vi "Edit_Raw_data_file_setups.vi"(4 "LDA set up":T1={"dimensions"=enum."2D", "Arrival spacing"=FALSE, "Sigma cut"=6, "Transit time"=FALSE, "Min time interval ms"=0.1} {"Min time interval ms" format="%.1f"}, 5 "LDA stats weighting":string, 6 "Raw data filename":path, 7 "Meas setup file":string="Colourimeter setup") -> ()   [LabVIEW 2010]
uses:
  Globals/Constants_global.vi
panel:
  out "Appended string":string
  out "Output string":string
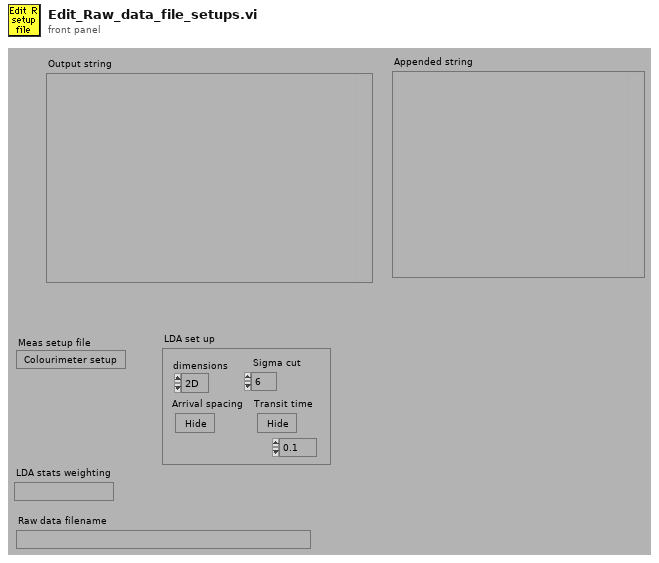
[diagram p1: front panel]
types:
  T1 = cluster{"dimensions":enum16{"1D", "2D"}, "Arrival spacing":bool, "Sigma cut":i32, "Transit time":bool, "Min time interval ms":dbl}
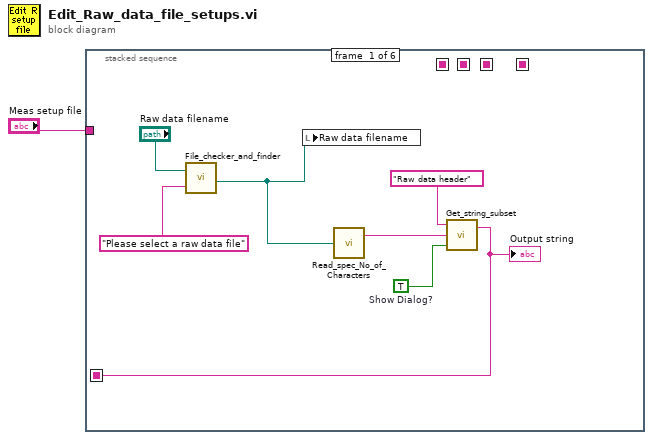
[diagram p0: block diagram]
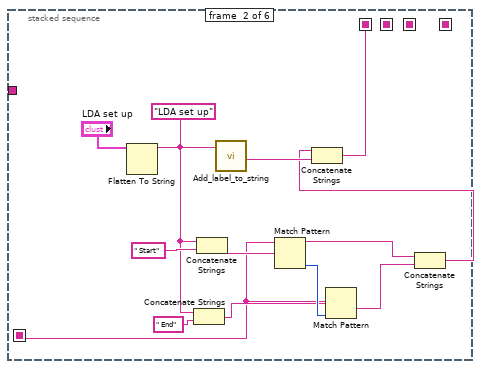
[diagram p2: hidden frame]
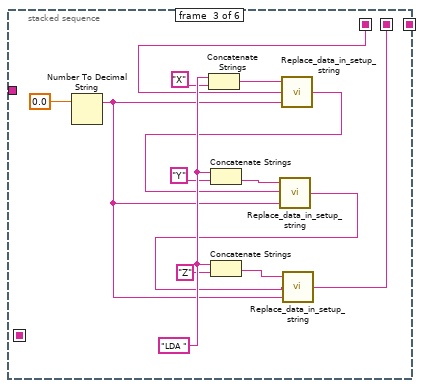
[diagram p3: hidden frame]
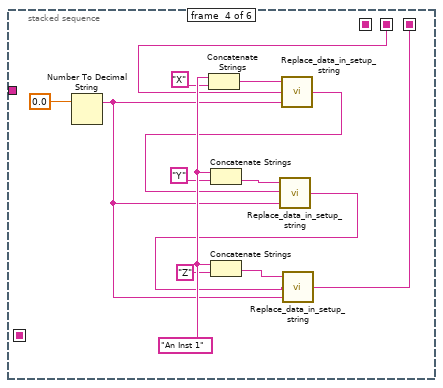
[diagram p4: hidden frame]
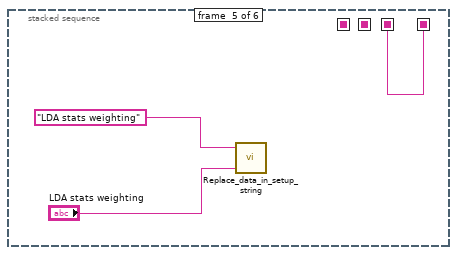
[diagram p5: hidden frame]
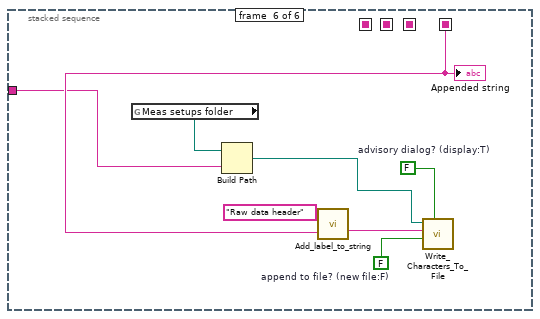
[diagram p6: hidden frame]
diagram:
  n1 = stacked-sequence {
    seq-local: [w7 _ _ _ _ _] -> [_ w12 _ _ _ _]
    seq-local: [_ _ _ w36 _ _] -> [_ _ _ _ w49 _]
    seq-local: [_ _ _ _ w49 _] -> [_ _ _ _ _ w55]
    seq-local: [_ w19 _ _ _ _] -> [_ _ w29 _ _ _]
    seq-local: [_ _ w23 _ _ _] -> [_ _ _ w37 _ _]
    tunnel: "Meas setup file" -> [_ _ _ _ _ w53]
    frame #0 {
      w2 = TRUE  # Show Dialog?
      n2 = call "File_checker_and_finder.vi"("Promp if not found"="Please select a raw data file", "Filename In"="Raw data filename") -> ("Filename Out"=w4:path)  [unwired: 1 out]
      n3 = local write "Raw data filename"(w4) -> ()
      n4 = call "Read_spec_No_of_Characters.vi"("Filename"=w4) -> ("character string"=w3:string)  [unwired: 1 out]
      n5 = call "Get_string_subset.vi"("Show Dialog?"=w2, "String to split"=w3, "File Label"="Raw data header") -> ("Output string"=w7:string)  [unwired: 1 out]
      "Output string" <- w7
    }
    frame #1 {
      w17 = "LDA set up" ("Label for characters")
      n6 = Flatten To String(anything="LDA set up") -> (data string=w22:string)  [unwired: 3 in, 2 out]
      n7 = Concatenate Strings(w17, " End" ("Output string")) -> (w13:string)
      n8 = Concatenate Strings(w17, " Start" ("Output string")) -> (w15:string)
      n9 = call "Add_label_to_string.vi"("String to write"=w22, "File Label"=w17) -> ("Output string"=w20:string)
      n10 = Match Pattern(string=w12, regular expression=w15) -> (before substring=w10:string, offset past match=w14:i32)  [unwired: 1 in, 2 out]
      n11 = Match Pattern(string=w12, regular expression=w13, offset (0)=w14) -> (after substring=w11:string)  [unwired: 3 out]
      n12 = Concatenate Strings(w10, w11) -> (w9:string)
      n13 = Concatenate Strings(w9, w20) -> (w19:string)
    }
    frame #2 {
      w35 = "LDA "
      n14 = Number To Decimal String(number=0.0) -> (decimal integer string=w24:string)  [unwired: 1 in]
      n15 = Concatenate Strings(w35, "X") -> (w31:string)
      n16 = Concatenate Strings(w35, "Y") -> (w27:string)
      n17 = Concatenate Strings(w35, "Z") -> (w28:string)
      n18 = call "Replace_data_in_setup_string.vi"("New data string"=w24, "Input string"=w29, "Variable name"=w31) -> ("Appended string"=w26:string)
      n19 = call "Replace_data_in_setup_string.vi"("New data string"=w24, "Input string"=w26, "Variable name"=w27) -> ("Appended string"=w25:string)
      n20 = call "Replace_data_in_setup_string.vi"("New data string"=w24, "Input string"=w25, "Variable name"=w28) -> ("Appended string"=w23:string)
    }
    frame #3 {
      w48 = "An Inst 1"
      n21 = Number To Decimal String(number=0.0) -> (decimal integer string=w38:string)  [unwired: 1 in]
      n22 = Concatenate Strings(w48, "X") -> (w44:string)
      n23 = Concatenate Strings(w48, "Y") -> (w41:string)
      n24 = Concatenate Strings(w48, "Z") -> (w42:string)
      n25 = call "Replace_data_in_setup_string.vi"("New data string"=w38, "Input string"=w37, "Variable name"=w44) -> ("Appended string"=w40:string)
      n26 = call "Replace_data_in_setup_string.vi"("New data string"=w38, "Input string"=w40, "Variable name"=w41) -> ("Appended string"=w39:string)
      n27 = call "Replace_data_in_setup_string.vi"("New data string"=w38, "Input string"=w39, "Variable name"=w42) -> ("Appended string"=w36:string)
    }
    frame #4 {
      n28 = call "Replace_data_in_setup_string.vi"("New data string"="LDA stats weighting", "Variable name"="LDA stats weighting") -> ()  [unwired: 1 in, 1 out]
    }
    frame #5 {
      w58 = FALSE  # advisory dialog? (display:T)
      w59 = FALSE  # append to file? (new file:F)
      n29 = global read "Constants_global.vi" "Meas setups folder"() -> (w54:path)
      n30 = Build Path(base path=w54, name or relative path=w53) -> (appended path=w52:path)
      n31 = call "Add_label_to_string.vi"("String to write"=w55, "File Label"="Raw data header") -> ("Output string"=w56:string)
      n32 = call "Write_Characters_To_File.vi"("file path (dialog if empty)"=w52, "advisory dialog? (display:T)"=w58, "character string"=w56, "append to file? (new file:F)"=w59) -> ()  [unwired: 4 in, 1 out]
      "Appended string" <- w55
    }
  }
